vi "Close Notifiers.vi"(8 "error in":errorcluster, 11 "Notifiers":T1) -> (0 "error out":errorcluster)   [LabVIEW 2017]
uses:
  Notifiers.ctl
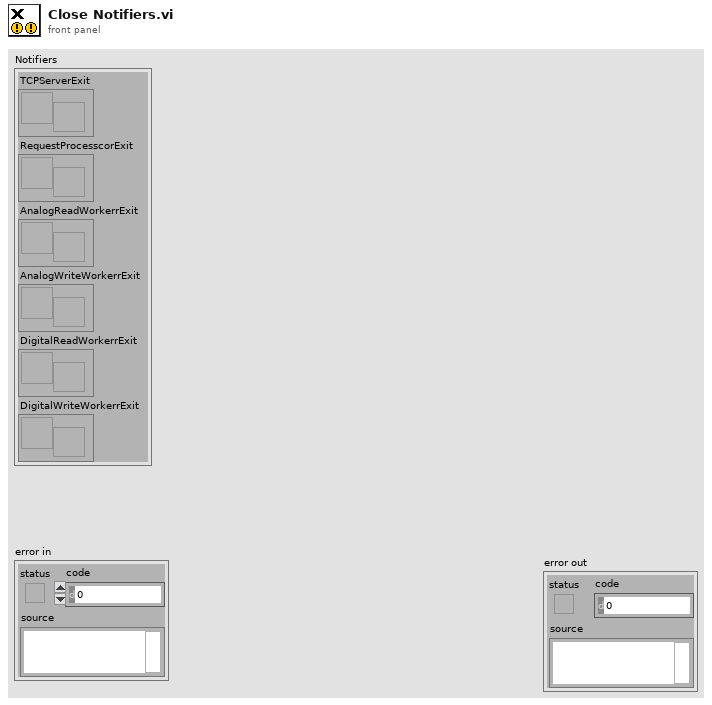
[diagram p1: front panel]
types:
  T1 = typedef "Notifiers.ctl" = cluster{"TCPServerExit":refnum<notifier>, "RequestProcesscorExit":refnum<notifier>, "AnalogReadWorkerrExit":refnum<notifier>, "AnalogWriteWorkerrExit":refnum<notifier>, "DigitalReadWorkerrExit":refnum<notifier>, "DigitalWriteWorkerrExit":refnum<notifier>}
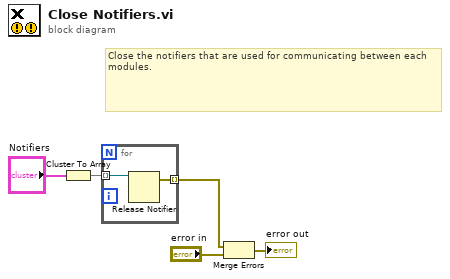
[diagram p0: block diagram]
diagram:
  # "Close the notifiers that are used for communicating between each modules."
  n1 = Cluster To Array(cluster="Notifiers") -> (array=w4:refnum<notifier>[])
  n2 = for {
    tunnel: w4 -> [w7] mode=indexing
    tunnel: [w6] -> w3 mode=indexing
    n3 = Release Notifier(notifier=w7) -> (error out=w6:errorcluster)  [unwired: 2 in, 2 out]
  }
  n4 = Merge Errors(w3, "error in") -> (→"error out":errorcluster)
